vi "Write contained configuration.vi"(8 "error in":errorcluster, 10 "module configuration":refnum<class "TBM module configuration.lvclass">, 11 "asynchronous execution module configuration in":refnum<class "asynchronous execution module configuration.lvclass">) -> (0 "error out":errorcluster, 3 "asynchronous execution module configuration out":refnum<class "asynchronous execution module configuration.lvclass">)   [LabVIEW 2013, in "asynchronous execution module configuration.lvclass"]
uses:
  asynchronous execution module configuration.lvclass
  <vilib>/NI/Tag Bus Module Framework/module configuration/TBM module configuration.lvclass
  asynchronous execution module configuration.lvclass/asynchronous execution module configuration.ctl
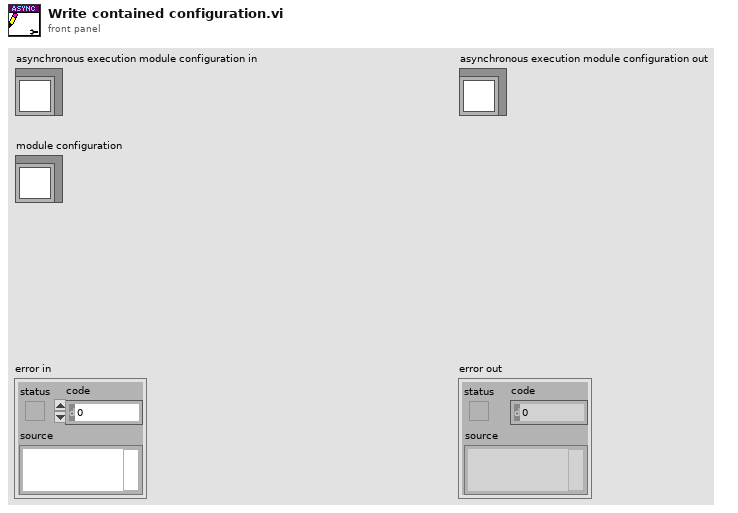
[diagram p1: front panel]
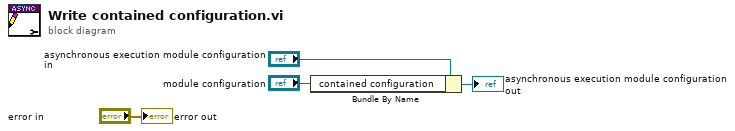
[diagram p0: block diagram]
diagram:
  n1 = Bundle By Name(cluster="asynchronous execution module configuration in", "contained configuration"="module configuration") -> (→"asynchronous execution module configuration out":refnum<class "asynchronous execution module configuration.lvclass">)
  "error out" <- "error in"
